vi "发送读取指定ID帧.vi"(0 "T_ID":u32, 5 "R_ID":u32, 7 "CAN_Frame":string, 9 "Time out(ms)":u32=500, 11 "error in (no error)":errorcluster, 12 "忽略接收":bool) -> (4 "OK":bool, 6 "Out_Time":bool, 8 "DataLen":u8, 10 "Recive":u8[](array[numeric]), 15 "error out":errorcluster)   [LabVIEW 2020]
uses:
  Global_Variable/Global.vi
  Libraries/ZLG_CAN/ZLG_CAN.lvlib
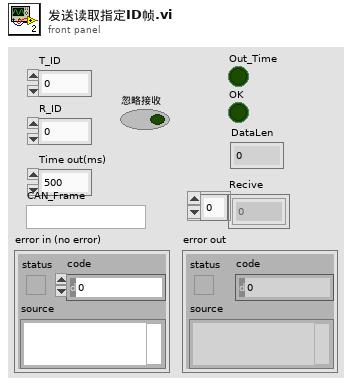
[diagram p1: front panel]
types:
  T1 = typedef "ZLG_CAN.lvlib/CAN_Frame.ctl" = cluster{"[0]":u8, "[1]":u8, "[2]":u8, "[3]":u8, "[4]":u8, "[5]":u8, "[6]":u8, "[7]":u8}
  T2 = typedef "ZLG_CAN.lvlib/Recive_Wait (Reply Payload)--cluster.ctl" = cluster{"Can_Receive":T3[], "Recive_Wait_error":errorcluster}
  T3 = typedef "ZLG_CAN.lvlib/CAN_OBJ_R.ctl" = cluster{"ID":u32, "TimeStamp":u32, "TimeFlag":u8, "SendType":u8, "RemoteFlag":u8, "ExternFlag":u8, "DataLen":u8, "数值":u8, "数值":u8, "数值":u8, "数值":u8, "数值":u8, "数值":u8, "数值":u8, "数值":u8, "数值":u8, "数值":u8, "数值":u8}
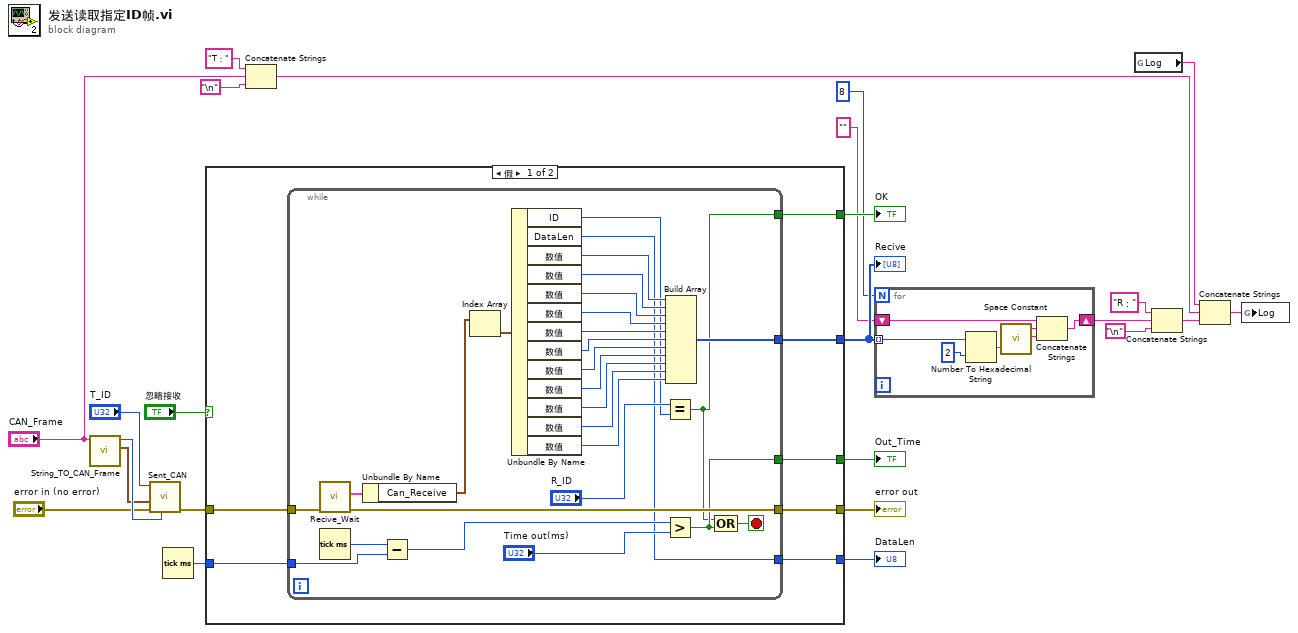
[diagram p0: block diagram]
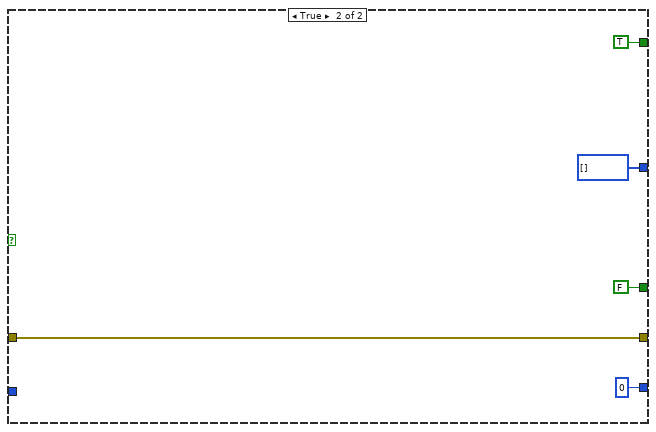
[diagram p2: hidden frame]
diagram:
  n1 = call "String_TO_CAN_Frame.vi"("CAN_Frame"="CAN_Frame") -> ("CAN_FRAME"=w23:T1, "DATA_LEN"=w24:i32)  [unwired: 9 in]
  n2 = call "Sent_CAN.vi"("帧长度"=w24, "error in (no error)"="error in (no error)", "帧数据"=w23, "ID"="T_ID") -> ("error out"=w22:errorcluster)  [unwired: 7 in]
  n3 = Tick Count (ms)() -> (millisecond timer value=w19:u32)
  n4 = case shown="假" "忽略接收" {
    tunnel: w22 -> [w31 w59]
    tunnel: w19 -> [w30 _]
    tunnel: [w29 w59] -> w18
    tunnel: [w28 u8 0 ("DataLen")] -> w17
    tunnel: [w27 FALSE] -> w16
    tunnel: [w26 TRUE] -> w15
    tunnel: [w25 u8[] []] -> w12
    frame False {
      n5 = while {
        tunnel: w31 -> [w56]
        tunnel: [w46] -> w25
        tunnel: w30 -> [w42]
        tunnel: [w39] -> w29
        tunnel: [w34] -> w28
        tunnel: [w33] -> w27
        tunnel: [w32] -> w26
        stop <- w44 stop-if-true
        n6 = call "Recive_Wait.vi"("error in (no error)"=w56) -> ("error out"=w39:errorcluster, "Reply Payload"=w55:T2)  [unwired: 8 in, 1 out]
        n7 = Tick Count (ms)() -> (millisecond timer value=w43:u32)
        n8 = Unbundle By Name(w55) -> ("Can_Receive"=w58:T3[])
        n9 = Subtract(x=w43, y=w42) -> (x-y=w41:u32)
        n10 = Index Array(array=w58) -> (element=w57:T3)  [unwired: 1 in]
        n11 = Unbundle By Name(w57) -> ("ID"=w35:u32, "DataLen"=w34:u8, "数值"=w54:u8, "数值"=w53:u8, "数值"=w52:u8, "数值"=w51:u8, "数值"=w50:u8, "数值"=w49:u8, "数值"=w48:u8, "数值"=w47:u8, "数值"=w38:u8, "数值"=w37:u8, "数值"=w36:u8)
        n12 = Equal?(x="R_ID", y=w35) -> (x = y?=w32:bool)
        n13 = Greater?(x=w41, y="Time out(ms)") -> (0:w33:bool)
        n14 = Build Array(w54, w53, w52, w51, w50, w49, w48, w47, w38, w37, w36) -> (w46:u8[])
        n15 = Compound Arithmetic op=OR ("复合运算")(w32, w33) -> (w44:bool)
      }
    }
    frame True {
    }
  }
  "Recive" <- w12
  "error out" <- w18
  "DataLen" <- w17
  "Out_Time" <- w16
  "OK" <- w15
  n16 = Concatenate Strings("T：" ("字符串"), "CAN_Frame", "\n") -> (w10:string)
  n17 = for {
    N: 8 -> [_]
    tunnel: w12 -> [w66] mode=indexing
    shift-right: [w68] -> w8
    shift-left: "" -> [w67]
    n18 = Number To Hexadecimal String(1:i16 2 ("宽度(-)"), 2:w66) -> (0:w64:string)
    n19 = call <vilib>:"Space Constant.vi"() -> ("String"=w69:string)
    n20 = Concatenate Strings(w67, w64, w69) -> (w68:string)
  }
  n21 = global read "Global.vi" "Log"() -> (w4:string)
  n22 = Concatenate Strings("R：" ("字符串"), w8, "\n") -> (w7:string)
  n23 = Concatenate Strings(w4, w10, w7) -> (w3:string)
  n24 = global write "Global.vi" "Log"(w3) -> ()
